vi "Unit Test.vi"() -> ()   [LabVIEW 2018]
uses:
  Custom Controls/System Units.ctl
  builds/Thermocouple.lvlibp/Thermocouple.lvclass
  Thermocouple.lvlib
panel:
  out "Temperature":dbl
  out "error out":errorcluster
  in  "SI":T1
  in  "error in":errorcluster
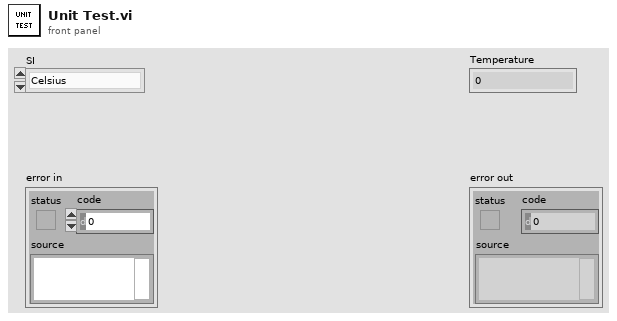
[diagram p1: front panel]
types:
  T1 = typedef "Thermocouple.lvlib/System Units.ctl" = enum16{"Celsius", "Fahrenheit"}
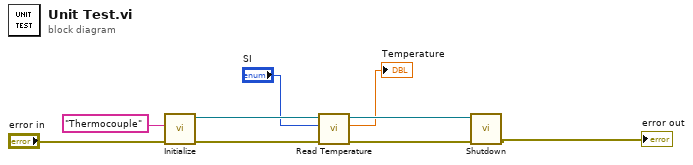
[diagram p0: block diagram]
diagram:
  n1 = call "Initialize.vi"("error in"="error in", "Device"="Thermocouple") -> ("error out"=w7:errorcluster, "Thermocouple out"=w6:refnum<class "Thermocouple.lvclass">)  [unwired: 8 in]
  n2 = call-dynamic "Read Temperature.vi"("error in (no error)"=w7, "SI"="SI", "Thermocouple in"=w6) -> ("error out"=w4:errorcluster, "Temperature"=→"Temperature":dbl, "Thermocouple out"=w5:refnum<class "Thermocouple.lvclass">)  [unwired: 6 in]
  n3 = call "Shutdown.vi"("error in (no error)"=w4, "Thermocouple in"=w5) -> ("error out"=→"error out":errorcluster)  [unwired: 8 in, 1 out]
